vi "Multi-camera acquisition of images.vi"() -> ()   [LabVIEW 2009]
uses:
  D/Program Files (x86)/National Instruments/LabVIEW 2015/user.lib/LabViewDVPCamera/LabViewDVPCamera.lvlib
panel:
  in  "CloseFlg 4":i32
  in  "CameraList 4":u16(ring) caption="CameraList" items=["USB2_1.2M_MONO(31)@UE121000026", "USB3_CMOS_16M(2)@UB16A000000"]
  in  "Set 4":bool
  in  "Open 4":bool
  in  "Close 4":bool
  in  "ScanCamera 4":bool
  out "handle 4":u32
  out "Image 4":T1(plugin-control)
  in  "CloseFlg 3":i32
  in  "CameraList 3":u16(ring) caption="CameraList" items=["USB2_1.2M_MONO(32)@UE121303030", "USB3_CMOS_16M(2)@UB16A000000"]
  in  "Set 3":bool
  in  "Open 3":bool
  in  "Close 3":bool
  in  "ScanCamera 3":bool
  out "handle 3":u32
  out "Image 3":T1(plugin-control)
  in  "CloseFlg 2":i32
  in  "CameraList 2":u16(ring) caption="CameraList" items=["USB2_1.2M_MONO(31)@UE121000026", "USB3_CMOS_16M(2)@UB16A000000"]
  in  "Set 2":bool
  in  "Open 2":bool
  in  "Close 2":bool
  in  "ScanCamera 2":bool
  out "handle 2":u32
  out "Image 2":T1(plugin-control)
  out "Image":T1(plugin-control)
  in  "CloseFlg":i32
  out "handle":u32
  in  "CameraList":u16(ring) items=["USB2_1.2M_MONO(32)@UE121303030", "USB3_CMOS_16M(2)@UB16A000000"]
  in  "Set":bool
  in  "Close":bool
  in  "Open":bool
  in  "ScanCamera":bool
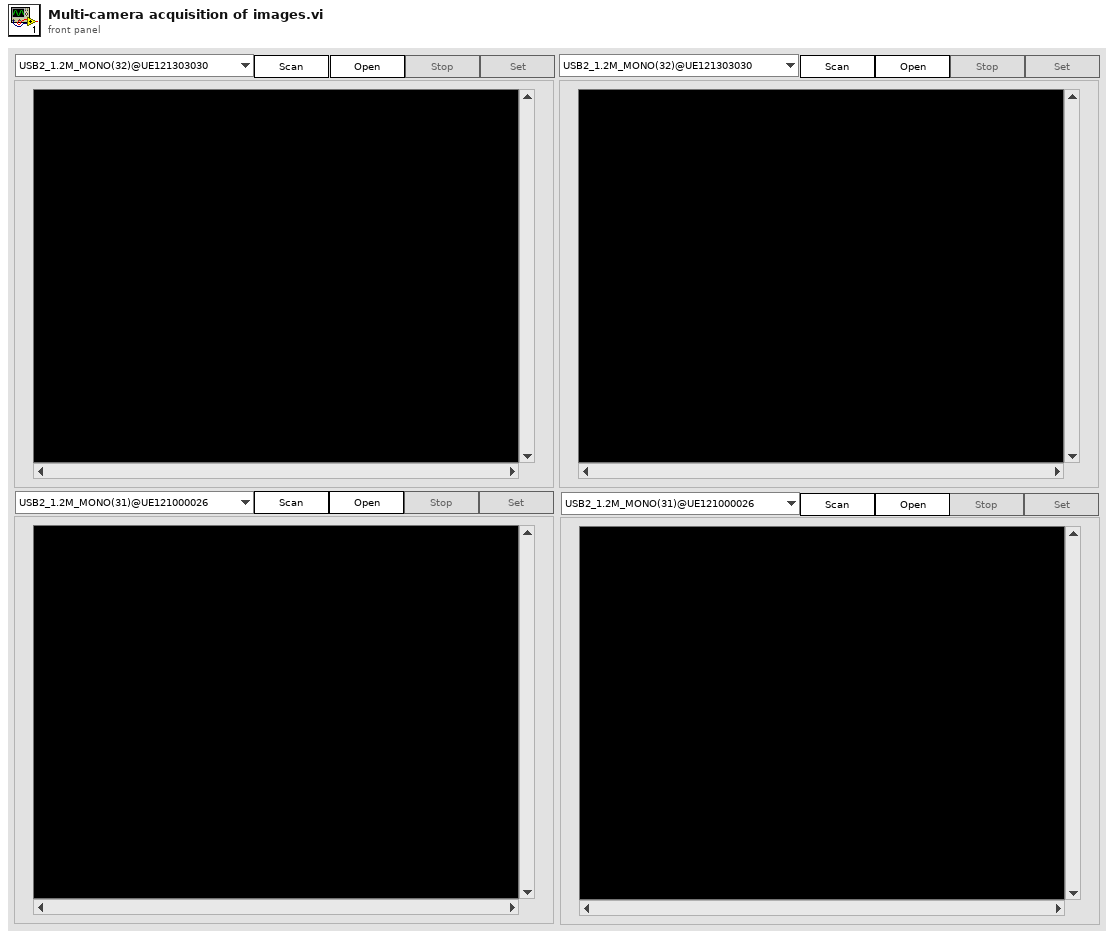
[diagram p1: front panel]
types:
  T1 = typedef "IMAQ Image.ctl" = refnum<image>
  T2 = enum8{"Enabled", "Disabled", "Disabled and Grayed Out"}
  T3 = typedef "LVStringsAndValuesArrayTypeDef_U16.ctl" = cluster{"String":string, "Value":u16}[]
  T4 = typedef "Image Type" = u32
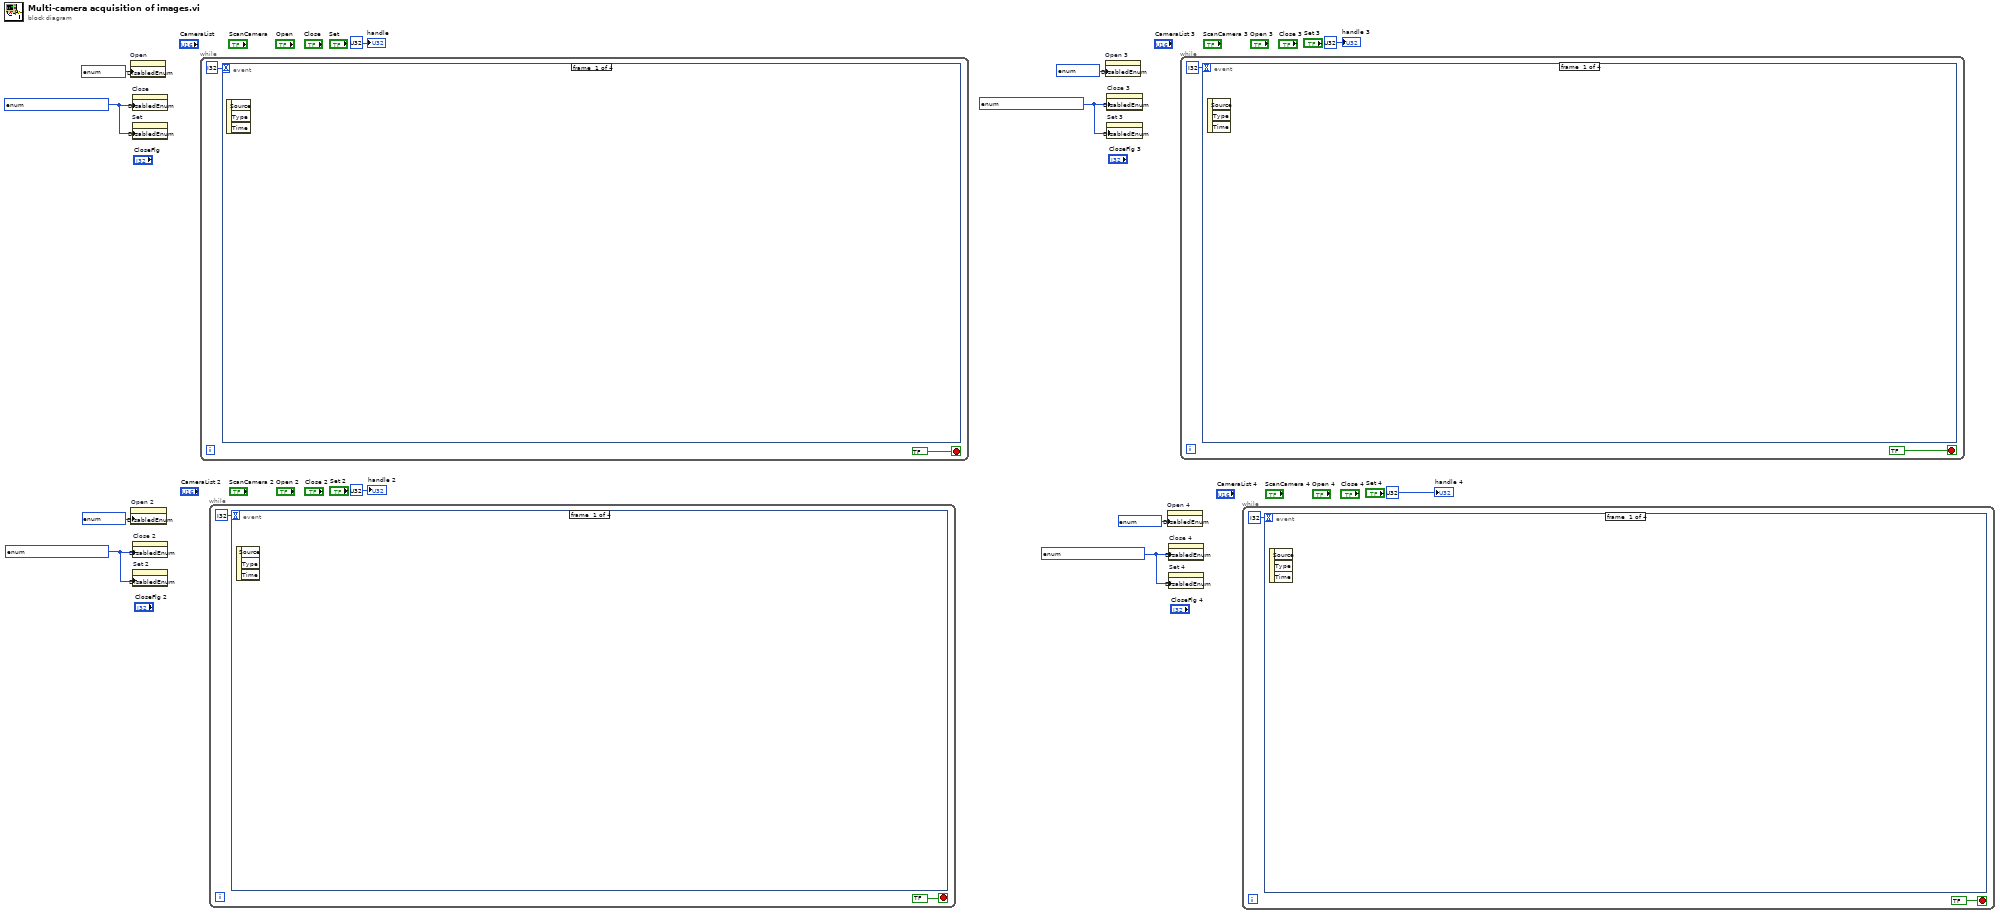
[diagram p0: block diagram]
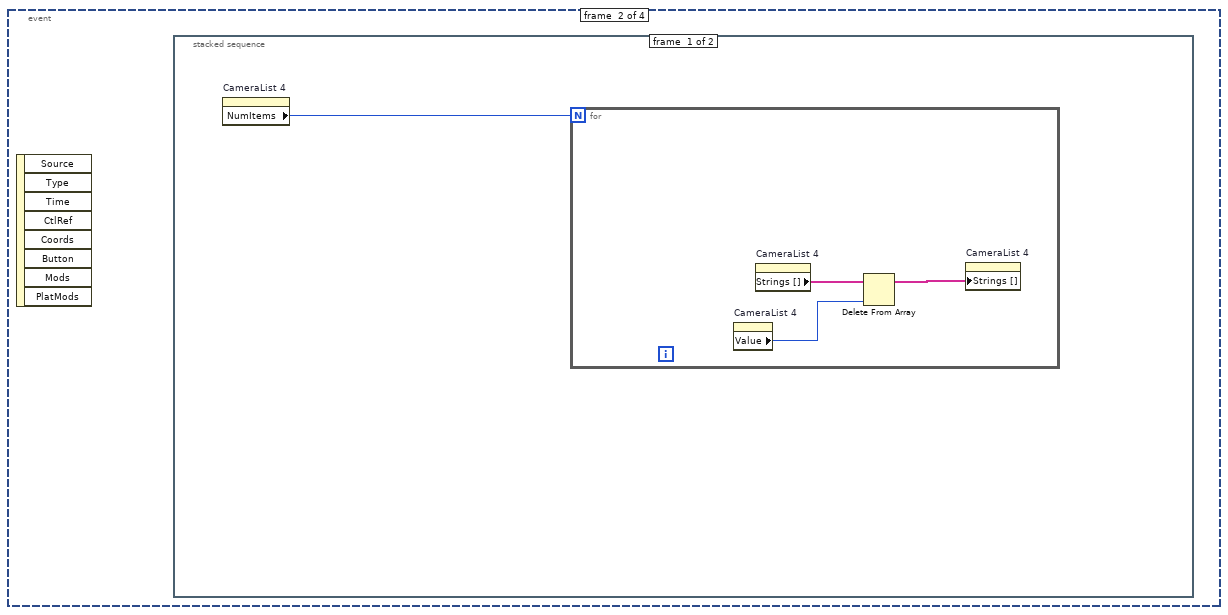
[diagram p2: hidden frame]
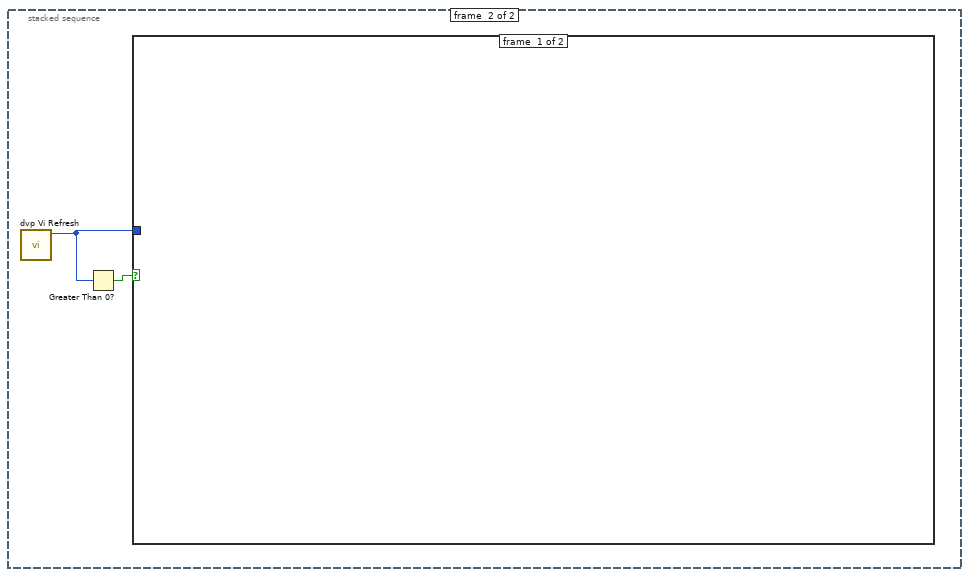
[diagram p3: hidden frame]
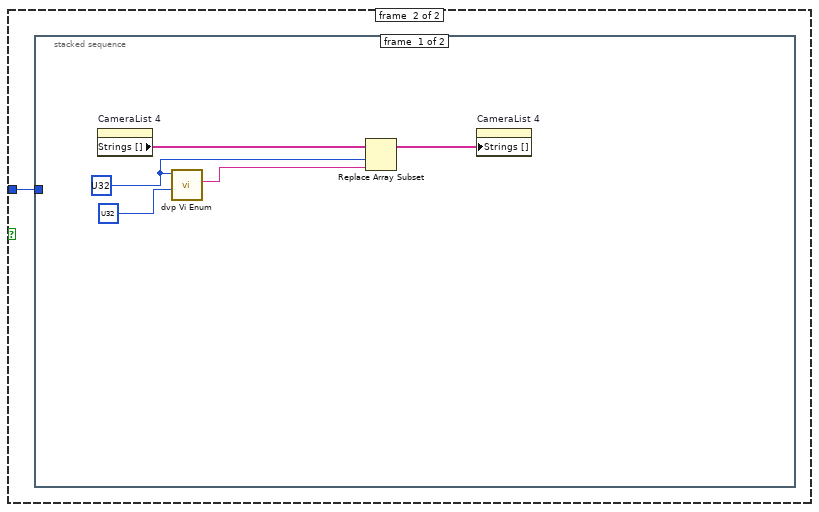
[diagram p4: hidden frame]
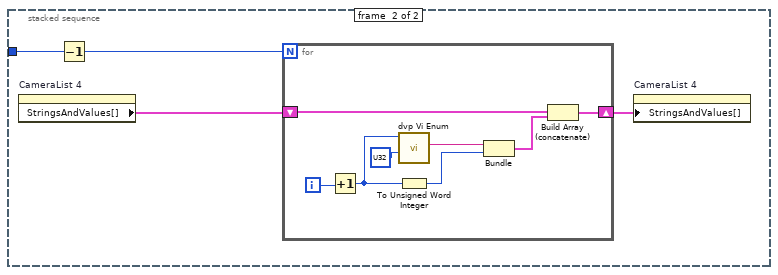
[diagram p5: hidden frame]
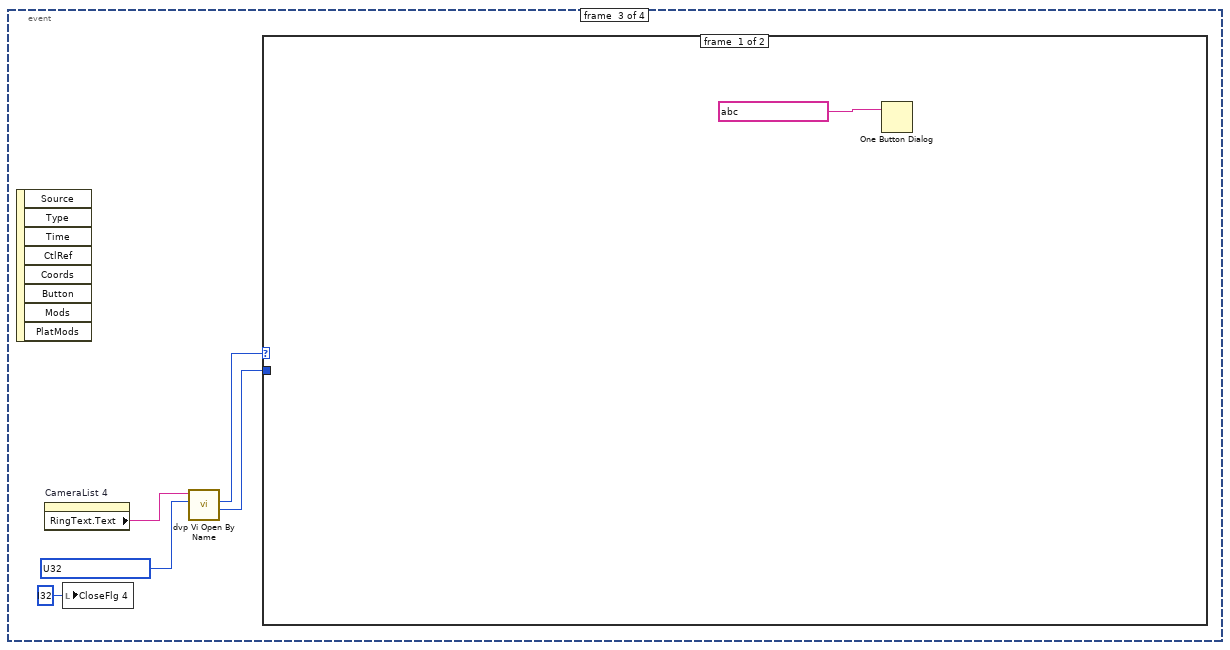
[diagram p6: hidden frame]
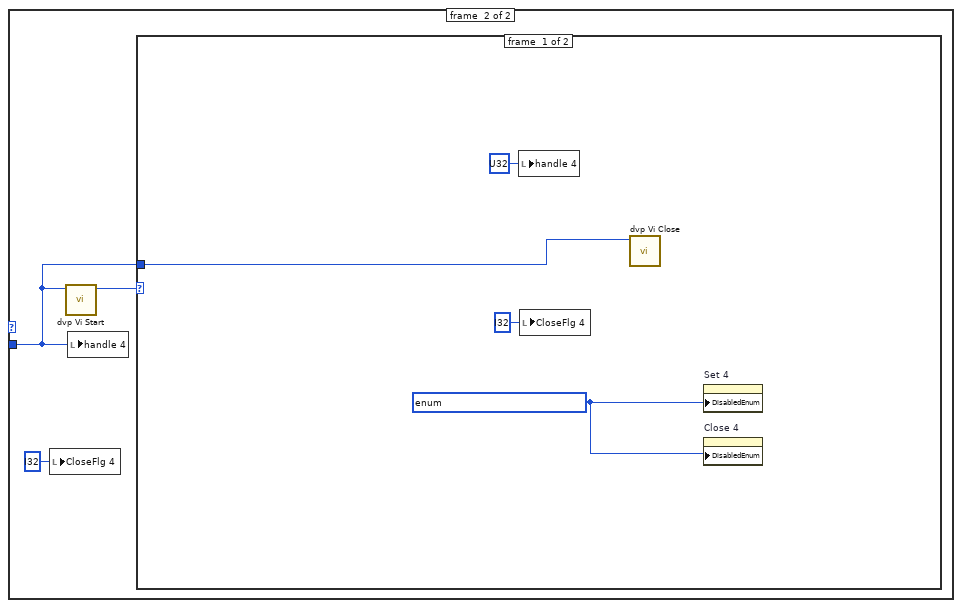
[diagram p7: hidden frame]
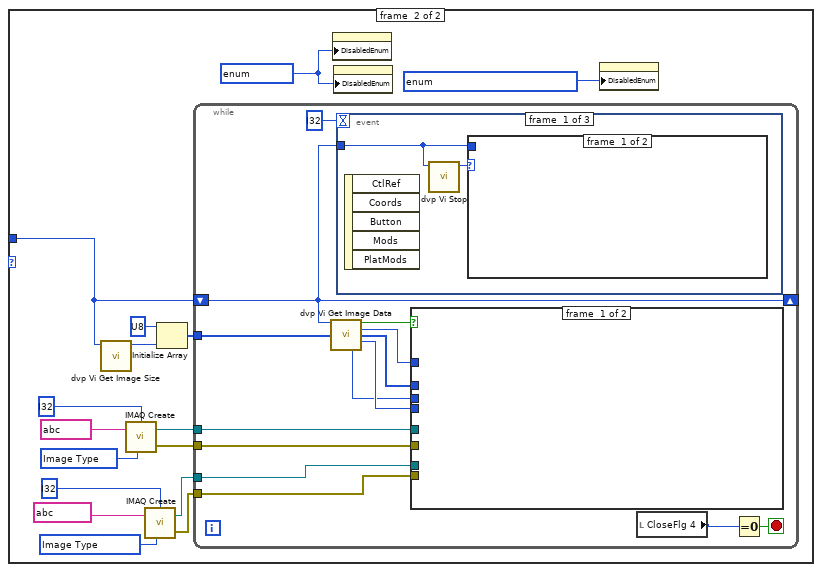
[diagram p8: hidden frame]
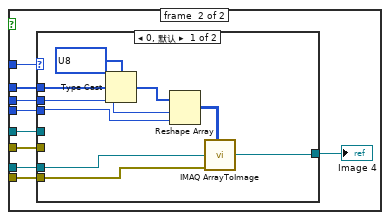
[diagram p9: hidden frame]
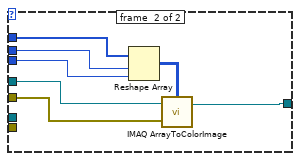
[diagram p10: hidden frame]
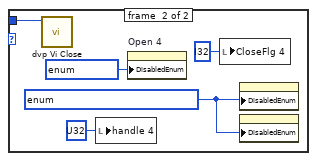
[diagram p11: hidden frame]
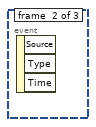
[diagram p12: hidden frame]
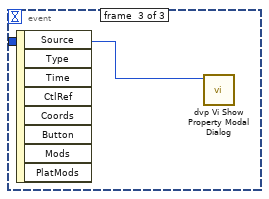
[diagram p13: hidden frame]
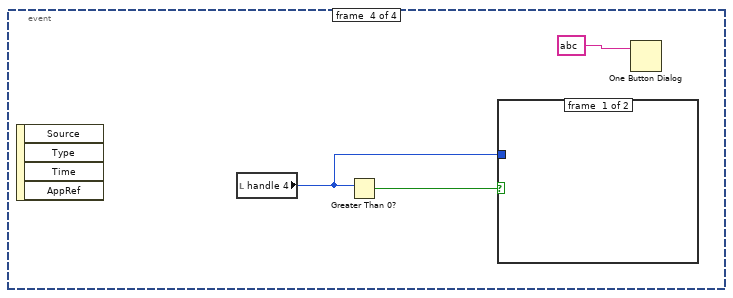
[diagram p14: hidden frame]
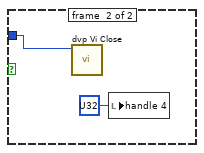
[diagram p15: hidden frame]
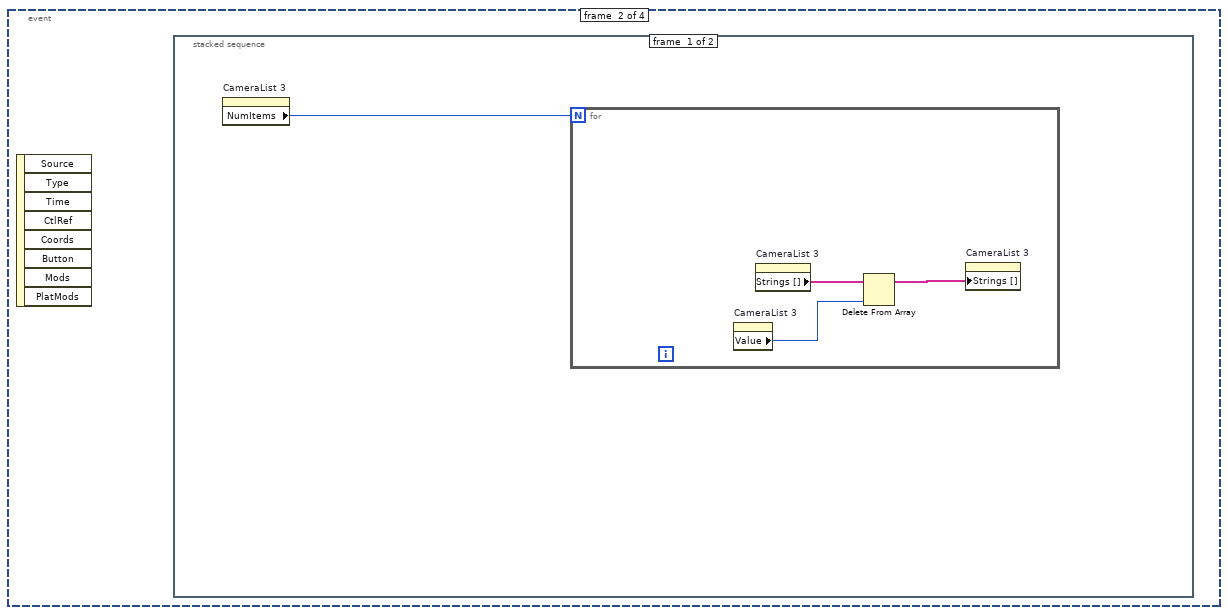
[diagram p16: hidden frame]
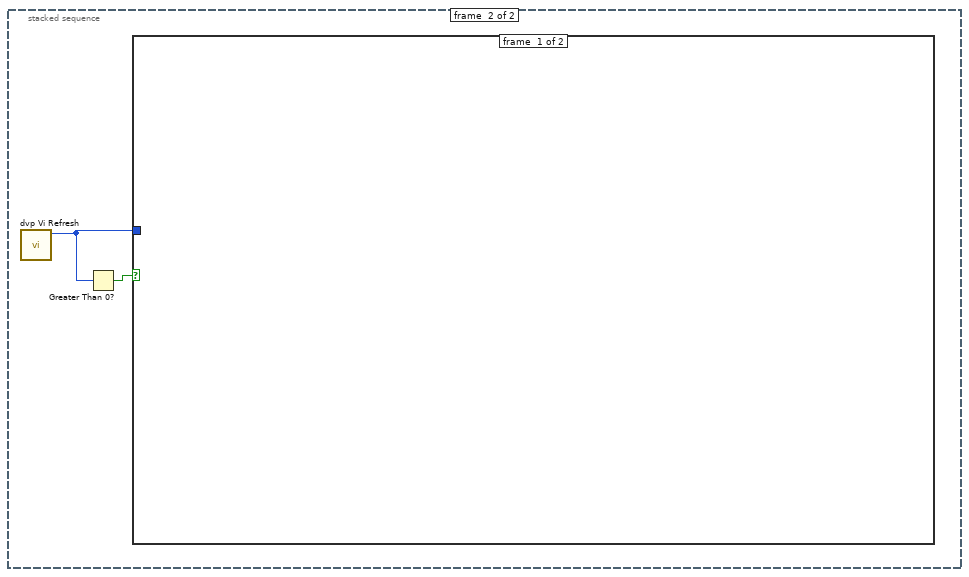
[diagram p17: hidden frame]
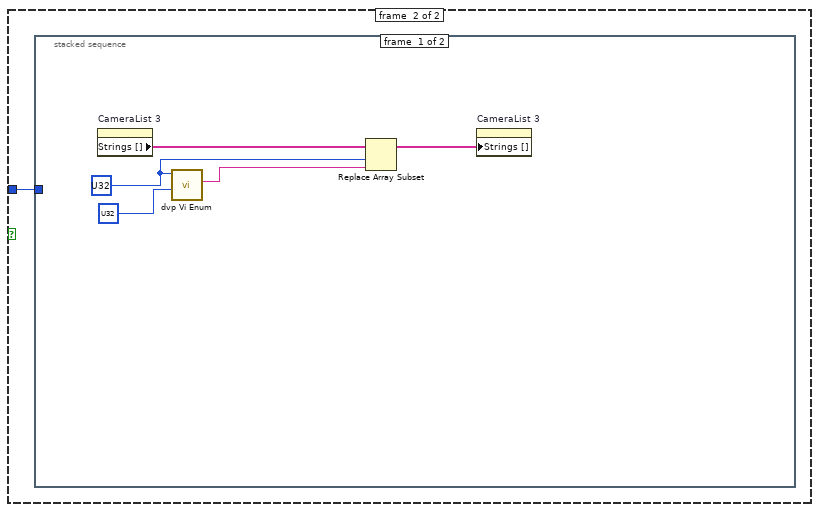
[diagram p18: hidden frame]
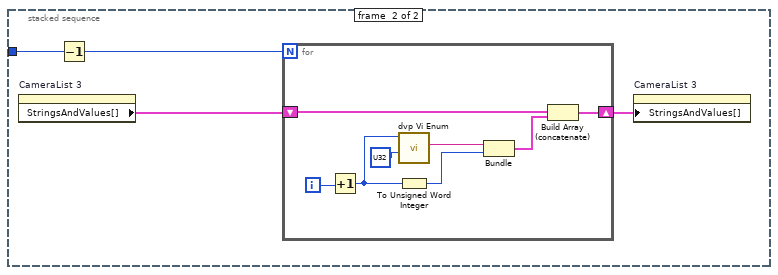
[diagram p19: hidden frame]
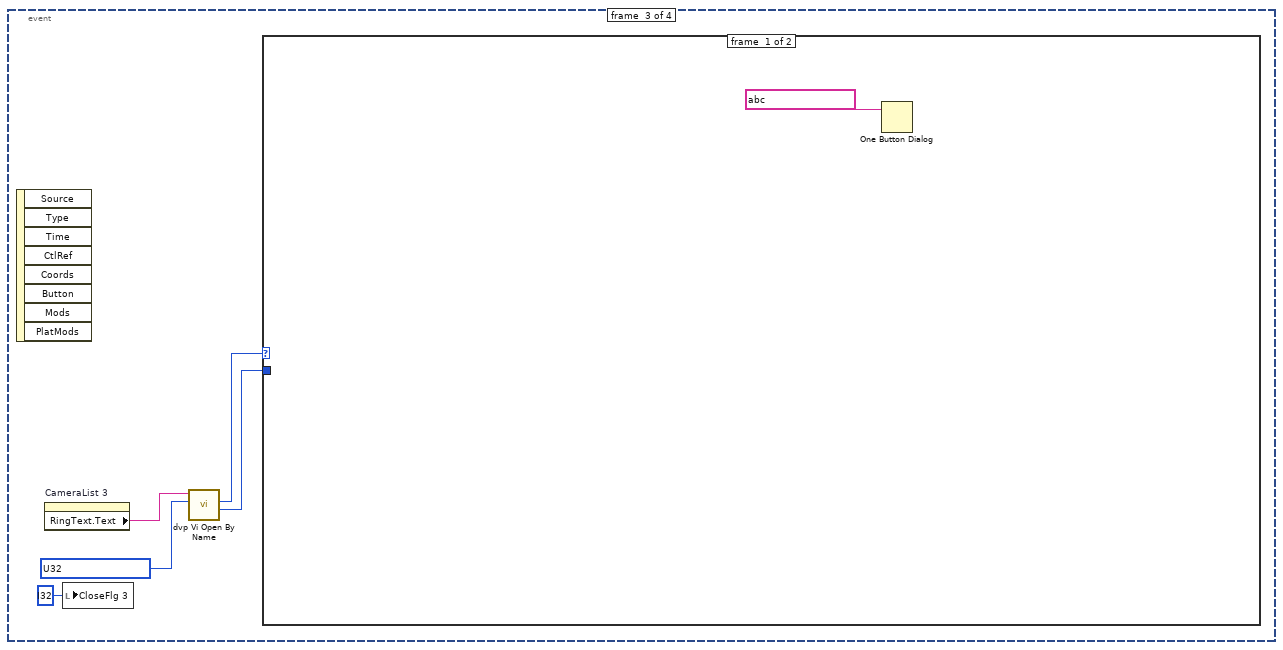
[diagram p20: hidden frame]
diagram:
  w2 = T2 ? ("禁用")
  w5 = T2 ? ("禁用")
  w8 = T2 ? ("禁用")
  w11 = T2 ? ("禁用")
  n1 = property on="Open" class="Bool"("DisabledEnum"=T2 ? ("禁用")) -> ()  [unwired: 2 in, 2 out]
  n2 = property on="Open 2" class="Bool"("DisabledEnum"=T2 ? ("禁用")) -> ()  [unwired: 2 in, 2 out]
  n3 = property on="Close" class="Bool"("DisabledEnum"=w11) -> ()  [unwired: 2 in, 2 out]
  n4 = property on="Set" class="Bool"("DisabledEnum"=w11) -> ()  [unwired: 2 in, 2 out]
  n5 = property on="Close 2" class="Bool"("DisabledEnum"=w8) -> ()  [unwired: 2 in, 2 out]
  n6 = property on="Set 2" class="Bool"("DisabledEnum"=w8) -> ()  [unwired: 2 in, 2 out]
  n7 = while {
    stop <- bool ? stop-if-true
    n8 = event shown="[2] \"Open\": 鼠标按下" {
      selector: _ -> [_ _ _ _]
      dyn-events: _ -> [_ _ _ _]
      timeout: i32 ? -> [_ _ _ _]
      event #0 {
        n9 = event-data() -> ()  [unwired: 1 in, 3 out]
      }
      event #1 {
        n10 = event-data() -> ()  [unwired: 1 in, 8 out]
        n11 = stacked-sequence "清除下拉列表的数据" {
          frame #0 {
            n12 = property on="CameraList" class="Ring (严格)"() -> ("NumItems"=w15:u32)  [unwired: 2 in, 2 out]
            n13 = for {
              N: w15 -> [_]
              n14 = property on="CameraList" class="Ring (严格)"() -> ("Value"=w17:u16)  [unwired: 2 in, 2 out]
              n15 = property on="CameraList" class="Ring (严格)"() -> ("Strings []"=w16:string[])  [unwired: 2 in, 2 out]
              n16 = Delete From Array ("删除数组元素")(array=w16, index=w17) -> (array with subset deleted=w18:string[])  [unwired: 1 in, 1 out]
              n17 = property on="CameraList" class="Ring (严格)"("Strings []"=w18) -> ()  [unwired: 2 in, 2 out]
            }
          }
          frame #1 {
            n18 = call "dvp Vi Refresh.vi"() -> ("pCount out"=w20:u32)  [unwired: 10 in, 1 out]
            n19 = Greater Than 0?(x=w20) -> (x > 0?=w19:bool)
            n20 = case shown="真" w19 {
              tunnel: w20 -> [_ w21]
              frame #0 {
              }
              frame #1 {
                n21 = stacked-sequence {
                  tunnel: w21 -> [_ w28]
                  frame #0 {
                    w22 = u32 ? ("index")
                    n22 = property on="CameraList" class="Ring (严格)"() -> ("Strings []"=w25:string[])  [unwired: 2 in, 2 out]
                    n23 = call "dvp Vi Enum.vi"("unSize"=u32 ?, "index"=w22) -> ("friendlyName out"=w24:string)  [unwired: 8 in, 1 out]
                    n24 = Replace Array Subset ("替换数组子集")(array=w25, new element=w24, index=w22) -> (w26:string[])
                    n25 = property on="CameraList" class="Ring (严格)"("Strings []"=w26) -> ()  [unwired: 2 in, 2 out]
                  }
                  frame #1 {
                    n26 = property on="CameraList" class="Ring (严格)"() -> ("StringsAndValues[]"=w30:T3)  [unwired: 2 in, 2 out]
                    n27 = Decrement(x=w28) -> (x-1=w27:u32)
                    n28 = for {
                      N: w27 -> [_]
                      shift-right: [w37] -> w29
                      shift-left: w30 -> [w35]
                      i -> [w32]
                      n29 = Increment(x=w32) -> (x+1=w31:i32)
                      n30 = call "dvp Vi Enum.vi"("unSize"=u32 ?, "index"=w31) -> ("friendlyName out"=w38:string)  [unwired: 8 in, 1 out]
                      n31 = To Unsigned Word Integer(number=w31) -> (unsigned 16bit integer=w34:u16)
                      n32 = Bundle("friendlyName out"=w38, w34) -> (w36:cluster{"friendlyName out":string, u16})  [unwired: 1 in]
                      n33 = Build Array (concatenate) ("创建数组")(w35, w36) -> (w37:T3)
                    }
                    n34 = property on="CameraList" class="Ring (严格)"("StringsAndValues[]"=w29) -> ()  [unwired: 2 in, 2 out]
                  }
                }
              }
            }
          }
        }
      }
      event #2 {
        w41 = u32 ? items=["OPEN_OFFLINE", "OPEN_NORMAL"] ("type")
        n35 = event-data() -> ()  [unwired: 1 in, 8 out]
        n36 = property on="CameraList" class="Ring (严格)"() -> ("RingText.Text"=w40:string)  [unwired: 2 in, 2 out]
        n37 = local write "CloseFlg"(i32 ? ("CloseFlg")) -> ()
        n38 = call "dvp Vi Open By Name.vi"("type"=w41, "friendlyName"=w40) -> ("pHandle out"=w43:u32, "function return"=w42:u32)  [unwired: 7 in, 1 out]
        n39 = case shown="1" w42 {
          tunnel: w43 -> [_ w47]
          frame #0 {
            n40 = One Button Dialog(message=string ? ("消息")) -> ()  [unwired: 1 in, 1 out]
          }
          frame #1 {
            n41 = call "dvp Vi Start.vi"("handle"=w47) -> ("function return"=w45:u32)  [unwired: 10 in]
            n42 = local write "handle"(w47) -> ()
            n43 = local write "CloseFlg"(i32 ? ("CloseFlg")) -> ()
            n44 = case shown="1" w45 {
              tunnel: w47 -> [w51 w63]
              frame #0 {
                w50 = T2 ? ("禁用")
                n45 = local write "handle"(u32 ? ("handle")) -> ()
                n46 = local write "CloseFlg"(i32 ? ("CloseFlg")) -> ()
                n47 = call "dvp Vi Close.vi"("handle"=w51) -> ()  [unwired: 10 in, 1 out]
                n48 = property on="Set" class="Bool"("DisabledEnum"=w50) -> ()  [unwired: 2 in, 2 out]
                n49 = property on="Close" class="Bool"("DisabledEnum"=w50) -> ()  [unwired: 2 in, 2 out]
              }
              frame #1 {
                w57 = T4 ? items=["Grayscale (U8)", "Grayscale (I16)", "Grayscale (SGL)", "Complex (CSG)", "RGB (U32)", "HSL (U32)", "RGB (U64)", "Grayscale (U16)"] ("Image Type")
                w61 = T4 ? items=["Grayscale (U8)", "Grayscale (I16)", "Grayscale (SGL)", "Complex (CSG)", "RGB (U32)", "HSL (U32)", "RGB (U64)", "Grayscale (U16)"] ("Image Type")
                w67 = T2 ? ("禁用")
                n50 = call "dvp Vi Get Image Size.vi"("handle"=w63) -> ("function return"=w62:u32)  [unwired: 10 in]
                n51 = call "IMAQ Create"("Border Size"=i32 ?, "Image Name"=string ?, "Image Type"=w61) -> ("New Image"=w56:T1, "error out"=w53:errorcluster)  [unwired: 2 in]
                n52 = call "IMAQ Create"("Border Size"=i32 ?, "Image Name"=string ?, "Image Type"=w57) -> ("New Image"=w55:T1, "error out"=w54:errorcluster)  [unwired: 2 in]
                n53 = Initialize Array(u8 ? ("元素"), w62) -> (w64:u8[])
                n54 = while {
                  shift-right: [w78] -> _
                  shift-left: w63 -> [w78]
                  tunnel: w64 -> [w77]
                  tunnel: w56 -> [w71]
                  tunnel: w55 -> [w70]
                  tunnel: w54 -> [w69]
                  tunnel: w53 -> [w68]
                  stop <- w80 stop-if-true
                  n55 = call "dvp Vi Get Image Data.vi"("handle"=w78, "pbuffer"=w77) -> ("piHeight out"=w75:i32, "function return"=w72:bool, "pformat out"=w73:i32, "pbuffer out"=w74:u32[], "piWidth out"=w76:i32)  [unwired: 9 in]
                  n56 = event shown="[0] \"Close\": 鼠标按下" {
                    selector: _ -> [_ _ _]
                    dyn-events: _ -> [_ _ _]
                    timeout: i32 ? -> [_ _ _]
                    tunnel: w78 -> [w107 _ w114]
                    event #0 {
                      n57 = event-data() -> ()  [unwired: 1 in, 5 out]
                      n58 = call "dvp Vi Stop.vi"("handle"=w107) -> ("function return"=w108:u32)  [unwired: 10 in]
                      n59 = case shown="1" w108 {
                        tunnel: w107 -> [_ w111]
                        frame #0 {
                        }
                        frame #1 {
                          w110 = T2 ? ("禁用")
                          n60 = call "dvp Vi Close.vi"("handle"=w111) -> ()  [unwired: 10 in, 1 out]
                          n61 = local write "handle"(u32 ? ("handle")) -> ()
                          n62 = property on="Open" class="Bool"("DisabledEnum"=T2 ? ("禁用")) -> ()  [unwired: 2 in, 2 out]
                          n63 = local write "CloseFlg"(i32 ? ("CloseFlg")) -> ()
                          n64 = property on="Close" class="Bool"("DisabledEnum"=w110) -> ()  [unwired: 2 in, 2 out]
                          n65 = property on="Set" class="Bool"("DisabledEnum"=w110) -> ()  [unwired: 2 in, 2 out]
                        }
                      }
                    }
                    event #1 {
                      n66 = event-data() -> ()  [unwired: 1 in, 3 out]
                    }
                    event #2 {
                      n67 = event-data() -> ()  [unwired: 1 in, 8 out]
                      n68 = call "dvp Vi Show Property Modal Dialog.vi"("handle"=w114) -> ()  [unwired: 10 in, 1 out]
                    }
                  }
                  n69 = case shown="真" w72 {
                    tunnel: w76 -> [_ w90]
                    tunnel: w75 -> [_ w89]
                    tunnel: w74 -> [_ w88]
                    tunnel: w73 -> [_ w87]
                    tunnel: w71 -> [_ w83]
                    tunnel: w70 -> [_ w86]
                    tunnel: w69 -> [_ w85]
                    tunnel: w68 -> [_ w84]
                    frame #0 {
                    }
                    frame #1 {
                      n70 = case shown="1" w87 {
                        tunnel: w89 -> [w99 w105]
                        tunnel: w90 -> [w98 w106]
                        tunnel: [w97 w103] -> w82
                        tunnel: w88 -> [w94 w102]
                        tunnel: w86 -> [w91 _]
                        tunnel: w85 -> [w92 _]
                        tunnel: w84 -> [_ w100]
                        tunnel: w83 -> [_ w101]
                        frame #0 {
                          n71 = Type Cast(type=u8[] ?, x=w94) -> (*(type *) &x=w93:u8[])
                          n72 = Reshape Array ("重排数组维数")(w93, w99, w98) -> (w96:u8[][])
                          n73 = call "IMAQ ArrayToImage"("error in (no error)"=w92, "Image Pixels (U8)"=w96, "Image"=w91) -> ("Image Out"=w97:T1)  [unwired: 7 in, 1 out]
                        }
                        frame #1 {
                          n74 = Reshape Array ("重排数组维数")(w102, w105, w106) -> (w104:u32[][])
                          n75 = call "IMAQ ArrayToColorImage"("Image Pixels (U32)"=w104, "Image"=w101, "error in (no error)"=w100) -> ("Image Out"=w103:T1)  [unwired: 2 in, 1 out]
                        }
                      }
                      "Image" <- w82
                    }
                  }
                  n76 = local read "CloseFlg"() -> (w79:i32)
                  n77 = Equal To 0?(x=w79) -> (x = 0?=w80:bool)
                }
                n78 = property on="Set" class="Bool"("DisabledEnum"=w67) -> ()  [unwired: 2 in, 2 out]
                n79 = property on="Close" class="Bool"("DisabledEnum"=w67) -> ()  [unwired: 2 in, 2 out]
                n80 = property on="Open" class="Bool"("DisabledEnum"=T2 ? ("禁用")) -> ()  [unwired: 2 in, 2 out]
              }
            }
          }
        }
      }
      event #3 {
        n81 = event-data() -> ()  [unwired: 1 in, 4 out]
        n82 = local read "handle"() -> (w115:u32)
        n83 = Greater Than 0?(x=w115) -> (x > 0?=w116:bool)
        n84 = case shown="真" w116 {
          tunnel: w115 -> [_ w119]
          frame #0 {
          }
          frame #1 {
            n85 = call "dvp Vi Close.vi"("handle"=w119) -> ()  [unwired: 10 in, 1 out]
            n86 = local write "handle"(u32 ? ("handle")) -> ()
          }
        }
        n87 = One Button Dialog(message=string ? ("消息")) -> ()  [unwired: 1 in, 1 out]
      }
    }
  }
  n88 = while {
    stop <- bool ? stop-if-true
    n89 = event shown="[2] \"Open 2\": 鼠标按下" {
      selector: _ -> [_ _ _ _]
      dyn-events: _ -> [_ _ _ _]
      timeout: i32 ? -> [_ _ _ _]
      event #0 {
        n90 = event-data() -> ()  [unwired: 1 in, 3 out]
      }
      event #1 {
        n91 = event-data() -> ()  [unwired: 1 in, 8 out]
        n92 = stacked-sequence "清除下拉列表的数据" {
          frame #0 {
            n93 = property on="CameraList 2" class="Ring (严格)"() -> ("NumItems"=w122:u32)  [unwired: 2 in, 2 out]
            n94 = for {
              N: w122 -> [_]
              n95 = property on="CameraList 2" class="Ring (严格)"() -> ("Value"=w124:u16)  [unwired: 2 in, 2 out]
              n96 = property on="CameraList 2" class="Ring (严格)"() -> ("Strings []"=w123:string[])  [unwired: 2 in, 2 out]
              n97 = Delete From Array ("删除数组元素")(array=w123, index=w124) -> (array with subset deleted=w125:string[])  [unwired: 1 in, 1 out]
              n98 = property on="CameraList 2" class="Ring (严格)"("Strings []"=w125) -> ()  [unwired: 2 in, 2 out]
            }
          }
          frame #1 {
            n99 = call "dvp Vi Refresh.vi"() -> ("pCount out"=w127:u32)  [unwired: 10 in, 1 out]
            n100 = Greater Than 0?(x=w127) -> (x > 0?=w126:bool)
            n101 = case shown="真" w126 {
              tunnel: w127 -> [_ w128]
              frame #0 {
              }
              frame #1 {
                n102 = stacked-sequence {
                  tunnel: w128 -> [_ w135]
                  frame #0 {
                    w129 = u32 ? ("index")
                    n103 = property on="CameraList 2" class="Ring (严格)"() -> ("Strings []"=w132:string[])  [unwired: 2 in, 2 out]
                    n104 = call "dvp Vi Enum.vi"("unSize"=u32 ?, "index"=w129) -> ("friendlyName out"=w131:string)  [unwired: 8 in, 1 out]
                    n105 = Replace Array Subset ("替换数组子集")(array=w132, new element=w131, index=w129) -> (w133:string[])
                    n106 = property on="CameraList 2" class="Ring (严格)"("Strings []"=w133) -> ()  [unwired: 2 in, 2 out]
                  }
                  frame #1 {
                    n107 = property on="CameraList 2" class="Ring (严格)"() -> ("StringsAndValues[]"=w137:T3)  [unwired: 2 in, 2 out]
                    n108 = Decrement(x=w135) -> (x-1=w134:u32)
                    n109 = for {
                      N: w134 -> [_]
                      shift-right: [w144] -> w136
                      shift-left: w137 -> [w142]
                      i -> [w139]
                      n110 = Increment(x=w139) -> (x+1=w138:i32)
                      n111 = call "dvp Vi Enum.vi"("unSize"=u32 ?, "index"=w138) -> ("friendlyName out"=w145:string)  [unwired: 8 in, 1 out]
                      n112 = To Unsigned Word Integer(number=w138) -> (unsigned 16bit integer=w141:u16)
                      n113 = Bundle("friendlyName out"=w145, w141) -> (w143:cluster{"friendlyName out":string, u16})  [unwired: 1 in]
                      n114 = Build Array (concatenate) ("创建数组")(w142, w143) -> (w144:T3)
                    }
                    n115 = property on="CameraList 2" class="Ring (严格)"("StringsAndValues[]"=w136) -> ()  [unwired: 2 in, 2 out]
                  }
                }
              }
            }
          }
        }
      }
      event #2 {
        w148 = u32 ? items=["OPEN_OFFLINE", "OPEN_NORMAL"] ("type")
        n116 = event-data() -> ()  [unwired: 1 in, 8 out]
        n117 = property on="CameraList 2" class="Ring (严格)"() -> ("RingText.Text"=w147:string)  [unwired: 2 in, 2 out]
        n118 = local write "CloseFlg 2"(i32 ? ("CloseFlg")) -> ()
        n119 = call "dvp Vi Open By Name.vi"("type"=w148, "friendlyName"=w147) -> ("pHandle out"=w150:u32, "function return"=w149:u32)  [unwired: 7 in, 1 out]
        n120 = case shown="1" w149 {
          tunnel: w150 -> [_ w154]
          frame #0 {
            n121 = One Button Dialog(message=string ? ("消息")) -> ()  [unwired: 1 in, 1 out]
          }
          frame #1 {
            n122 = local write "CloseFlg 2"(i32 ? ("CloseFlg")) -> ()
            n123 = call "dvp Vi Start.vi"("handle"=w154) -> ("function return"=w152:u32)  [unwired: 10 in]
            n124 = local write "handle 2"(w154) -> ()
            n125 = case shown="1" w152 {
              tunnel: w154 -> [w158 w170]
              frame #0 {
                w157 = T2 ? ("禁用")
                n126 = local write "handle 2"(u32 ? ("handle")) -> ()
                n127 = local write "CloseFlg 2"(i32 ? ("CloseFlg")) -> ()
                n128 = call "dvp Vi Close.vi"("handle"=w158) -> ()  [unwired: 10 in, 1 out]
                n129 = property on="Set 2" class="Bool"("DisabledEnum"=w157) -> ()  [unwired: 2 in, 2 out]
                n130 = property on="Close 2" class="Bool"("DisabledEnum"=w157) -> ()  [unwired: 2 in, 2 out]
              }
              frame #1 {
                w165 = T4 ? items=["Grayscale (U8)", "Grayscale (I16)", "Grayscale (SGL)", "Complex (CSG)", "RGB (U32)", "HSL (U32)", "RGB (U64)", "Grayscale (U16)"] ("Image Type")
                w168 = T4 ? items=["Grayscale (U8)", "Grayscale (I16)", "Grayscale (SGL)", "Complex (CSG)", "RGB (U32)", "HSL (U32)", "RGB (U64)", "Grayscale (U16)"] ("Image Type")
                w174 = T2 ? ("禁用")
                n131 = call "dvp Vi Get Image Size.vi"("handle"=w170) -> ("function return"=w169:u32)  [unwired: 10 in]
                n132 = call "IMAQ Create"("Border Size"=i32 ?, "Image Name"=string ?, "Image Type"=w165) -> ("New Image"=w162:T1, "error out"=w161:errorcluster)  [unwired: 2 in]
                n133 = call "IMAQ Create"("Border Size"=i32 ?, "Image Name"=string ?, "Image Type"=w168) -> ("New Image"=w160:T1, "error out"=w159:errorcluster)  [unwired: 2 in]
                n134 = Initialize Array(u8 ? ("元素"), w169) -> (w171:u8[])
                n135 = while {
                  shift-right: [w185] -> _
                  shift-left: w170 -> [w185]
                  tunnel: w171 -> [w184]
                  tunnel: w162 -> [w178]
                  tunnel: w161 -> [w177]
                  tunnel: w160 -> [w176]
                  tunnel: w159 -> [w175]
                  stop <- w187 stop-if-true
                  n136 = call "dvp Vi Get Image Data.vi"("handle"=w185, "pbuffer"=w184) -> ("piHeight out"=w182:i32, "function return"=w179:bool, "pformat out"=w180:i32, "pbuffer out"=w181:u32[], "piWidth out"=w183:i32)  [unwired: 9 in]
                  n137 = event shown="[2] \"Set 2\": 鼠标按下" {
                    selector: _ -> [_ _ _]
                    dyn-events: _ -> [_ _ _]
                    timeout: i32 ? -> [_ _ _]
                    tunnel: w185 -> [w214 _ w221]
                    event #0 {
                      n138 = event-data() -> ()  [unwired: 1 in, 5 out]
                      n139 = call "dvp Vi Stop.vi"("handle"=w214) -> ("function return"=w215:u32)  [unwired: 10 in]
                      n140 = case shown="1" w215 {
                        tunnel: w214 -> [_ w218]
                        frame #0 {
                        }
                        frame #1 {
                          w217 = T2 ? ("禁用")
                          n141 = call "dvp Vi Close.vi"("handle"=w218) -> ()  [unwired: 10 in, 1 out]
                          n142 = local write "handle 2"(u32 ? ("handle")) -> ()
                          n143 = property on="Open 2" class="Bool"("DisabledEnum"=T2 ? ("禁用")) -> ()  [unwired: 2 in, 2 out]
                          n144 = local write "CloseFlg 2"(i32 ? ("CloseFlg")) -> ()
                          n145 = property on="Close 2" class="Bool"("DisabledEnum"=w217) -> ()  [unwired: 2 in, 2 out]
                          n146 = property on="Set 2" class="Bool"("DisabledEnum"=w217) -> ()  [unwired: 2 in, 2 out]
                        }
                      }
                    }
                    event #1 {
                      n147 = event-data() -> ()  [unwired: 1 in, 3 out]
                    }
                    event #2 {
                      n148 = event-data() -> ()  [unwired: 1 in, 8 out]
                      n149 = call "dvp Vi Show Property Modal Dialog.vi"("handle"=w221) -> ()  [unwired: 10 in, 1 out]
                    }
                  }
                  n150 = case shown="真" w179 {
                    tunnel: w183 -> [_ w197]
                    tunnel: w182 -> [_ w196]
                    tunnel: w181 -> [_ w194]
                    tunnel: w180 -> [_ w193]
                    tunnel: w178 -> [_ w192]
                    tunnel: w177 -> [_ w191]
                    tunnel: w176 -> [_ w190]
                    tunnel: w175 -> [_ w189]
                    frame #0 {
                    }
                    frame #1 {
                      n151 = case shown="0, 默认" w193 {
                        tunnel: w196 -> [w206 w212]
                        tunnel: w197 -> [w205 w213]
                        tunnel: [w204 w210] -> w195
                        tunnel: w194 -> [w201 w209]
                        tunnel: w192 -> [_ w208]
                        tunnel: w191 -> [_ w207]
                        tunnel: w190 -> [w198 _]
                        tunnel: w189 -> [w199 _]
                        frame #0 {
                          n152 = Type Cast(type=u8[] ?, x=w201) -> (*(type *) &x=w200:u8[])
                          n153 = Reshape Array ("重排数组维数")(w200, w206, w205) -> (w203:u8[][])
                          n154 = call "IMAQ ArrayToImage"("error in (no error)"=w199, "Image Pixels (U8)"=w203, "Image"=w198) -> ("Image Out"=w204:T1)  [unwired: 7 in, 1 out]
                        }
                        frame #1 {
                          n155 = Reshape Array ("重排数组维数")(w209, w212, w213) -> (w211:u32[][])
                          n156 = call "IMAQ ArrayToColorImage"("Image Pixels (U32)"=w211, "Image"=w208, "error in (no error)"=w207) -> ("Image Out"=w210:T1)  [unwired: 2 in, 1 out]
                        }
                      }
                      "Image 2" <- w195
                    }
                  }
                  n157 = local read "CloseFlg 2"() -> (w186:i32)
                  n158 = Equal To 0?(x=w186) -> (x = 0?=w187:bool)
                }
                n159 = property on="Set 2" class="Bool"("DisabledEnum"=w174) -> ()  [unwired: 2 in, 2 out]
                n160 = property on="Close 2" class="Bool"("DisabledEnum"=w174) -> ()  [unwired: 2 in, 2 out]
                n161 = property on="Open 2" class="Bool"("DisabledEnum"=T2 ? ("禁用")) -> ()  [unwired: 2 in, 2 out]
              }
            }
          }
        }
      }
      event #3 {
        n162 = event-data() -> ()  [unwired: 1 in, 4 out]
        n163 = local read "handle 2"() -> (w222:u32)
        n164 = Greater Than 0?(x=w222) -> (x > 0?=w223:bool)
        n165 = case shown="真" w223 {
          tunnel: w222 -> [_ w226]
          frame #0 {
          }
          frame #1 {
            n166 = call "dvp Vi Close.vi"("handle"=w226) -> ()  [unwired: 10 in, 1 out]
            n167 = local write "handle 2"(u32 ? ("handle")) -> ()
          }
        }
        n168 = One Button Dialog(message=string ? ("消息")) -> ()  [unwired: 1 in, 1 out]
      }
    }
  }
  n169 = property on="Open 3" class="Bool"("DisabledEnum"=T2 ? ("禁用")) -> ()  [unwired: 2 in, 2 out]
  n170 = property on="Close 3" class="Bool"("DisabledEnum"=w5) -> ()  [unwired: 2 in, 2 out]
  n171 = property on="Set 3" class="Bool"("DisabledEnum"=w5) -> ()  [unwired: 2 in, 2 out]
  n172 = property on="Open 4" class="Bool"("DisabledEnum"=T2 ? ("禁用")) -> ()  [unwired: 2 in, 2 out]
  n173 = property on="Close 4" class="Bool"("DisabledEnum"=w2) -> ()  [unwired: 2 in, 2 out]
  n174 = property on="Set 4" class="Bool"("DisabledEnum"=w2) -> ()  [unwired: 2 in, 2 out]
  n175 = while {
    stop <- bool ? stop-if-true
    n176 = event shown="[1] \"ScanCamera 3\": 鼠标按下" {
      selector: _ -> [_ _ _ _]
      dyn-events: _ -> [_ _ _ _]
      timeout: i32 ? -> [_ _ _ _]
      event #0 {
        n177 = event-data() -> ()  [unwired: 1 in, 3 out]
      }
      event #1 {
        n178 = event-data() -> ()  [unwired: 1 in, 8 out]
        n179 = stacked-sequence "清除下拉列表的数据" {
          frame #0 {
            n180 = property on="CameraList 3" class="Ring (严格)"() -> ("NumItems"=w229:u32)  [unwired: 2 in, 2 out]
            n181 = for {
              N: w229 -> [_]
              n182 = property on="CameraList 3" class="Ring (严格)"() -> ("Value"=w231:u16)  [unwired: 2 in, 2 out]
              n183 = property on="CameraList 3" class="Ring (严格)"() -> ("Strings []"=w230:string[])  [unwired: 2 in, 2 out]
              n184 = Delete From Array ("删除数组元素")(array=w230, index=w231) -> (array with subset deleted=w232:string[])  [unwired: 1 in, 1 out]
              n185 = property on="CameraList 3" class="Ring (严格)"("Strings []"=w232) -> ()  [unwired: 2 in, 2 out]
            }
          }
          frame #1 {
            n186 = call "dvp Vi Refresh.vi"() -> ("pCount out"=w234:u32)  [unwired: 10 in, 1 out]
            n187 = Greater Than 0?(x=w234) -> (x > 0?=w233:bool)
            n188 = case shown="真" w233 {
              tunnel: w234 -> [_ w235]
              frame #0 {
              }
              frame #1 {
                n189 = stacked-sequence {
                  tunnel: w235 -> [_ w242]
                  frame #0 {
                    w236 = u32 ? ("index")
                    n190 = property on="CameraList 3" class="Ring (严格)"() -> ("Strings []"=w239:string[])  [unwired: 2 in, 2 out]
                    n191 = call "dvp Vi Enum.vi"("unSize"=u32 ?, "index"=w236) -> ("friendlyName out"=w238:string)  [unwired: 8 in, 1 out]
                    n192 = Replace Array Subset ("替换数组子集")(array=w239, new element=w238, index=w236) -> (w240:string[])
                    n193 = property on="CameraList 3" class="Ring (严格)"("Strings []"=w240) -> ()  [unwired: 2 in, 2 out]
                  }
                  frame #1 {
                    n194 = property on="CameraList 3" class="Ring (严格)"() -> ("StringsAndValues[]"=w244:T3)  [unwired: 2 in, 2 out]
                    n195 = Decrement(x=w242) -> (x-1=w241:u32)
                    n196 = for {
                      N: w241 -> [_]
                      shift-right: [w251] -> w243
                      shift-left: w244 -> [w249]
                      i -> [w246]
                      n197 = Increment(x=w246) -> (x+1=w245:i32)
                      n198 = call "dvp Vi Enum.vi"("unSize"=u32 ?, "index"=w245) -> ("friendlyName out"=w252:string)  [unwired: 8 in, 1 out]
                      n199 = To Unsigned Word Integer(number=w245) -> (unsigned 16bit integer=w248:u16)
                      n200 = Bundle("friendlyName out"=w252, w248) -> (w250:cluster{"friendlyName out":string, u16})  [unwired: 1 in]
                      n201 = Build Array (concatenate) ("创建数组")(w249, w250) -> (w251:T3)
                    }
                    n202 = property on="CameraList 3" class="Ring (严格)"("StringsAndValues[]"=w243) -> ()  [unwired: 2 in, 2 out]
                  }
                }
              }
            }
          }
        }
      }
      event #2 {
        w255 = u32 ? items=["OPEN_OFFLINE", "OPEN_NORMAL"] ("type")
        n203 = event-data() -> ()  [unwired: 1 in, 8 out]
        n204 = property on="CameraList 3" class="Ring (严格)"() -> ("RingText.Text"=w254:string)  [unwired: 2 in, 2 out]
        n205 = local write "CloseFlg 3"(i32 ? ("CloseFlg")) -> ()
        n206 = call "dvp Vi Open By Name.vi"("type"=w255, "friendlyName"=w254) -> ("pHandle out"=w257:u32, "function return"=w256:u32)  [unwired: 7 in, 1 out]
        n207 = case shown="1" w256 {
          tunnel: w257 -> [_ w261]
          frame #0 {
            n208 = One Button Dialog(message=string ? ("消息")) -> ()  [unwired: 1 in, 1 out]
          }
          frame #1 {
            n209 = local write "CloseFlg 3"(i32 ? ("CloseFlg")) -> ()
            n210 = call "dvp Vi Start.vi"("handle"=w261) -> ("function return"=w259:u32)  [unwired: 10 in]
            n211 = local write "handle 3"(w261) -> ()
            n212 = case shown="1" w259 {
              tunnel: w261 -> [w265 w277]
              frame #0 {
                w264 = T2 ? ("禁用")
                n213 = local write "handle 3"(u32 ? ("handle")) -> ()
                n214 = local write "CloseFlg 3"(i32 ? ("CloseFlg")) -> ()
                n215 = call "dvp Vi Close.vi"("handle"=w265) -> ()  [unwired: 10 in, 1 out]
                n216 = property on="Set 3" class="Bool"("DisabledEnum"=w264) -> ()  [unwired: 2 in, 2 out]
                n217 = property on="Close 3" class="Bool"("DisabledEnum"=w264) -> ()  [unwired: 2 in, 2 out]
              }
              frame #1 {
                w273 = T4 ? items=["Grayscale (U8)", "Grayscale (I16)", "Grayscale (SGL)", "Complex (CSG)", "RGB (U32)", "HSL (U32)", "RGB (U64)", "Grayscale (U16)"] ("Image Type")
                w275 = T4 ? items=["Grayscale (U8)", "Grayscale (I16)", "Grayscale (SGL)", "Complex (CSG)", "RGB (U32)", "HSL (U32)", "RGB (U64)", "Grayscale (U16)"] ("Image Type")
                w281 = T2 ? ("禁用")
                n218 = call "dvp Vi Get Image Size.vi"("handle"=w277) -> ("function return"=w276:u32)  [unwired: 10 in]
                n219 = call "IMAQ Create"("Border Size"=i32 ?, "Image Name"=string ?, "Image Type"=w275) -> ("New Image"=w267:T1, "error out"=w266:errorcluster)  [unwired: 2 in]
                n220 = call "IMAQ Create"("Border Size"=i32 ?, "Image Name"=string ?, "Image Type"=w273) -> ("New Image"=w269:T1, "error out"=w268:errorcluster)  [unwired: 2 in]
                n221 = Initialize Array(u8 ? ("元素"), w276) -> (w278:u8[])
                n222 = while {
                  shift-right: [w292] -> _
                  shift-left: w277 -> [w292]
                  tunnel: w278 -> [w291]
                  tunnel: w269 -> [w285]
                  tunnel: w268 -> [w284]
                  tunnel: w267 -> [w283]
                  tunnel: w266 -> [w282]
                  stop <- w294 stop-if-true
                  n223 = call "dvp Vi Get Image Data.vi"("handle"=w292, "pbuffer"=w291) -> ("piHeight out"=w289:i32, "function return"=w286:bool, "pformat out"=w287:i32, "pbuffer out"=w288:u32[], "piWidth out"=w290:i32)  [unwired: 9 in]
                  n224 = event shown="[2] \"Set 3\": 鼠标按下" {
                    selector: _ -> [_ _ _]
                    dyn-events: _ -> [_ _ _]
                    timeout: i32 ? -> [_ _ _]
                    tunnel: w292 -> [w321 _ w328]
                    event #0 {
                      n225 = event-data() -> ()  [unwired: 1 in, 5 out]
                      n226 = call "dvp Vi Stop.vi"("handle"=w321) -> ("function return"=w322:u32)  [unwired: 10 in]
                      n227 = case shown="1" w322 {
                        tunnel: w321 -> [_ w325]
                        frame #0 {
                        }
                        frame #1 {
                          w324 = T2 ? ("禁用")
                          n228 = call "dvp Vi Close.vi"("handle"=w325) -> ()  [unwired: 10 in, 1 out]
                          n229 = local write "handle 3"(u32 ? ("handle")) -> ()
                          n230 = property on="Open 3" class="Bool"("DisabledEnum"=T2 ? ("禁用")) -> ()  [unwired: 2 in, 2 out]
                          n231 = local write "CloseFlg 3"(i32 ? ("CloseFlg")) -> ()
                          n232 = property on="Close 3" class="Bool"("DisabledEnum"=w324) -> ()  [unwired: 2 in, 2 out]
                          n233 = property on="Set 3" class="Bool"("DisabledEnum"=w324) -> ()  [unwired: 2 in, 2 out]
                        }
                      }
                    }
                    event #1 {
                      n234 = event-data() -> ()  [unwired: 1 in, 3 out]
                    }
                    event #2 {
                      n235 = event-data() -> ()  [unwired: 1 in, 8 out]
                      n236 = call "dvp Vi Show Property Modal Dialog.vi"("handle"=w328) -> ()  [unwired: 10 in, 1 out]
                    }
                  }
                  n237 = case shown="真" w286 {
                    tunnel: w290 -> [_ w304]
                    tunnel: w289 -> [_ w303]
                    tunnel: w288 -> [_ w302]
                    tunnel: w287 -> [_ w301]
                    tunnel: w285 -> [_ w300]
                    tunnel: w284 -> [_ w299]
                    tunnel: w283 -> [_ w298]
                    tunnel: w282 -> [_ w297]
                    frame #0 {
                    }
                    frame #1 {
                      n238 = case shown="1" w301 {
                        tunnel: w303 -> [w313 w319]
                        tunnel: w304 -> [w312 w320]
                        tunnel: [w311 w317] -> w296
                        tunnel: w302 -> [w308 w316]
                        tunnel: w300 -> [w306 _]
                        tunnel: w299 -> [w305 _]
                        tunnel: w298 -> [_ w315]
                        tunnel: w297 -> [_ w314]
                        frame #0 {
                          n239 = Type Cast(type=u8[] ?, x=w308) -> (*(type *) &x=w307:u8[])
                          n240 = Reshape Array ("重排数组维数")(w307, w313, w312) -> (w310:u8[][])
                          n241 = call "IMAQ ArrayToImage"("error in (no error)"=w305, "Image Pixels (U8)"=w310, "Image"=w306) -> ("Image Out"=w311:T1)  [unwired: 7 in, 1 out]
                        }
                        frame #1 {
                          n242 = Reshape Array ("重排数组维数")(w316, w319, w320) -> (w318:u32[][])
                          n243 = call "IMAQ ArrayToColorImage"("Image Pixels (U32)"=w318, "Image"=w315, "error in (no error)"=w314) -> ("Image Out"=w317:T1)  [unwired: 2 in, 1 out]
                        }
                      }
                      "Image 3" <- w296
                    }
                  }
                  n244 = local read "CloseFlg 3"() -> (w293:i32)
                  n245 = Equal To 0?(x=w293) -> (x = 0?=w294:bool)
                }
                n246 = property on="Set 3" class="Bool"("DisabledEnum"=w281) -> ()  [unwired: 2 in, 2 out]
                n247 = property on="Close 3" class="Bool"("DisabledEnum"=w281) -> ()  [unwired: 2 in, 2 out]
                n248 = property on="Open 3" class="Bool"("DisabledEnum"=T2 ? ("禁用")) -> ()  [unwired: 2 in, 2 out]
              }
            }
          }
        }
      }
      event #3 {
        n249 = event-data() -> ()  [unwired: 1 in, 4 out]
        n250 = local read "handle 3"() -> (w329:u32)
        n251 = Greater Than 0?(x=w329) -> (x > 0?=w330:bool)
        n252 = case shown="真" w330 {
          tunnel: w329 -> [_ w333]
          frame #0 {
          }
          frame #1 {
            n253 = call "dvp Vi Close.vi"("handle"=w333) -> ()  [unwired: 10 in, 1 out]
            n254 = local write "handle 3"(u32 ? ("handle")) -> ()
          }
        }
        n255 = One Button Dialog(message=string ? ("消息")) -> ()  [unwired: 1 in, 1 out]
      }
    }
  }
  n256 = while {
    stop <- bool ? stop-if-true
    n257 = event shown="[2] \"Open 4\": 鼠标按下" {
      selector: _ -> [_ _ _ _]
      dyn-events: _ -> [_ _ _ _]
      timeout: i32 ? -> [_ _ _ _]
      event #0 {
        n258 = event-data() -> ()  [unwired: 1 in, 3 out]
      }
      event #1 {
        n259 = event-data() -> ()  [unwired: 1 in, 8 out]
        n260 = stacked-sequence "清除下拉列表的数据" {
          frame #0 {
            n261 = property on="CameraList 4" class="Ring (严格)"() -> ("NumItems"=w336:u32)  [unwired: 2 in, 2 out]
            n262 = for {
              N: w336 -> [_]
              n263 = property on="CameraList 4" class="Ring (严格)"() -> ("Value"=w338:u16)  [unwired: 2 in, 2 out]
              n264 = property on="CameraList 4" class="Ring (严格)"() -> ("Strings []"=w337:string[])  [unwired: 2 in, 2 out]
              n265 = Delete From Array ("删除数组元素")(array=w337, index=w338) -> (array with subset deleted=w339:string[])  [unwired: 1 in, 1 out]
              n266 = property on="CameraList 4" class="Ring (严格)"("Strings []"=w339) -> ()  [unwired: 2 in, 2 out]
            }
          }
          frame #1 {
            n267 = call "dvp Vi Refresh.vi"() -> ("pCount out"=w341:u32)  [unwired: 10 in, 1 out]
            n268 = Greater Than 0?(x=w341) -> (x > 0?=w340:bool)
            n269 = case shown="真" w340 {
              tunnel: w341 -> [_ w342]
              frame #0 {
              }
              frame #1 {
                n270 = stacked-sequence {
                  tunnel: w342 -> [_ w349]
                  frame #0 {
                    w343 = u32 ? ("index")
                    n271 = property on="CameraList 4" class="Ring (严格)"() -> ("Strings []"=w346:string[])  [unwired: 2 in, 2 out]
                    n272 = call "dvp Vi Enum.vi"("unSize"=u32 ?, "index"=w343) -> ("friendlyName out"=w345:string)  [unwired: 8 in, 1 out]
                    n273 = Replace Array Subset ("替换数组子集")(array=w346, new element=w345, index=w343) -> (w347:string[])
                    n274 = property on="CameraList 4" class="Ring (严格)"("Strings []"=w347) -> ()  [unwired: 2 in, 2 out]
                  }
                  frame #1 {
                    n275 = property on="CameraList 4" class="Ring (严格)"() -> ("StringsAndValues[]"=w351:T3)  [unwired: 2 in, 2 out]
                    n276 = Decrement(x=w349) -> (x-1=w348:u32)
                    n277 = for {
                      N: w348 -> [_]
                      shift-right: [w358] -> w350
                      shift-left: w351 -> [w356]
                      i -> [w353]
                      n278 = Increment(x=w353) -> (x+1=w352:i32)
                      n279 = call "dvp Vi Enum.vi"("unSize"=u32 ?, "index"=w352) -> ("friendlyName out"=w359:string)  [unwired: 8 in, 1 out]
                      n280 = To Unsigned Word Integer(number=w352) -> (unsigned 16bit integer=w355:u16)
                      n281 = Bundle("friendlyName out"=w359, w355) -> (w357:cluster{"friendlyName out":string, u16})  [unwired: 1 in]
                      n282 = Build Array (concatenate) ("创建数组")(w356, w357) -> (w358:T3)
                    }
                    n283 = property on="CameraList 4" class="Ring (严格)"("StringsAndValues[]"=w350) -> ()  [unwired: 2 in, 2 out]
                  }
                }
              }
            }
          }
        }
      }
      event #2 {
        w362 = u32 ? items=["OPEN_OFFLINE", "OPEN_NORMAL"] ("type")
        n284 = event-data() -> ()  [unwired: 1 in, 8 out]
        n285 = property on="CameraList 4" class="Ring (严格)"() -> ("RingText.Text"=w361:string)  [unwired: 2 in, 2 out]
        n286 = local write "CloseFlg 4"(i32 ? ("CloseFlg")) -> ()
        n287 = call "dvp Vi Open By Name.vi"("type"=w362, "friendlyName"=w361) -> ("pHandle out"=w364:u32, "function return"=w363:u32)  [unwired: 7 in, 1 out]
        n288 = case shown="1" w363 {
          tunnel: w364 -> [_ w368]
          frame #0 {
            n289 = One Button Dialog(message=string ? ("消息")) -> ()  [unwired: 1 in, 1 out]
          }
          frame #1 {
            n290 = local write "CloseFlg 4"(i32 ? ("CloseFlg")) -> ()
            n291 = call "dvp Vi Start.vi"("handle"=w368) -> ("function return"=w366:u32)  [unwired: 10 in]
            n292 = local write "handle 4"(w368) -> ()
            n293 = case shown="1" w366 {
              tunnel: w368 -> [w372 w384]
              frame #0 {
                w371 = T2 ? ("禁用")
                n294 = local write "handle 4"(u32 ? ("handle")) -> ()
                n295 = local write "CloseFlg 4"(i32 ? ("CloseFlg")) -> ()
                n296 = call "dvp Vi Close.vi"("handle"=w372) -> ()  [unwired: 10 in, 1 out]
                n297 = property on="Set 4" class="Bool"("DisabledEnum"=w371) -> ()  [unwired: 2 in, 2 out]
                n298 = property on="Close 4" class="Bool"("DisabledEnum"=w371) -> ()  [unwired: 2 in, 2 out]
              }
              frame #1 {
                w379 = T4 ? items=["Grayscale (U8)", "Grayscale (I16)", "Grayscale (SGL)", "Complex (CSG)", "RGB (U32)", "HSL (U32)", "RGB (U64)", "Grayscale (U16)"] ("Image Type")
                w382 = T4 ? items=["Grayscale (U8)", "Grayscale (I16)", "Grayscale (SGL)", "Complex (CSG)", "RGB (U32)", "HSL (U32)", "RGB (U64)", "Grayscale (U16)"] ("Image Type")
                w388 = T2 ? ("禁用")
                n299 = call "dvp Vi Get Image Size.vi"("handle"=w384) -> ("function return"=w383:u32)  [unwired: 10 in]
                n300 = call "IMAQ Create"("Border Size"=i32 ?, "Image Name"=string ?, "Image Type"=w379) -> ("New Image"=w376:T1, "error out"=w375:errorcluster)  [unwired: 2 in]
                n301 = call "IMAQ Create"("Border Size"=i32 ?, "Image Name"=string ?, "Image Type"=w382) -> ("New Image"=w374:T1, "error out"=w373:errorcluster)  [unwired: 2 in]
                n302 = Initialize Array(u8 ? ("元素"), w383) -> (w385:u8[])
                n303 = while {
                  shift-right: [w399] -> _
                  shift-left: w384 -> [w399]
                  tunnel: w385 -> [w398]
                  tunnel: w376 -> [w392]
                  tunnel: w375 -> [w391]
                  tunnel: w374 -> [w390]
                  tunnel: w373 -> [w389]
                  stop <- w401 stop-if-true
                  n304 = call "dvp Vi Get Image Data.vi"("handle"=w399, "pbuffer"=w398) -> ("piHeight out"=w396:i32, "function return"=w393:bool, "pformat out"=w394:i32, "pbuffer out"=w395:u32[], "piWidth out"=w397:i32)  [unwired: 9 in]
                  n305 = event shown="[2] \"Set 4\": 鼠标按下" {
                    selector: _ -> [_ _ _]
                    dyn-events: _ -> [_ _ _]
                    timeout: i32 ? -> [_ _ _]
                    tunnel: w399 -> [w428 _ w435]
                    event #0 {
                      n306 = event-data() -> ()  [unwired: 1 in, 5 out]
                      n307 = call "dvp Vi Stop.vi"("handle"=w428) -> ("function return"=w429:u32)  [unwired: 10 in]
                      n308 = case shown="1" w429 {
                        tunnel: w428 -> [_ w432]
                        frame #0 {
                        }
                        frame #1 {
                          w431 = T2 ? ("禁用")
                          n309 = call "dvp Vi Close.vi"("handle"=w432) -> ()  [unwired: 10 in, 1 out]
                          n310 = local write "handle 4"(u32 ? ("handle")) -> ()
                          n311 = property on="Open 4" class="Bool"("DisabledEnum"=T2 ? ("禁用")) -> ()  [unwired: 2 in, 2 out]
                          n312 = local write "CloseFlg 4"(i32 ? ("CloseFlg")) -> ()
                          n313 = property on="Close 4" class="Bool"("DisabledEnum"=w431) -> ()  [unwired: 2 in, 2 out]
                          n314 = property on="Set 4" class="Bool"("DisabledEnum"=w431) -> ()  [unwired: 2 in, 2 out]
                        }
                      }
                    }
                    event #1 {
                      n315 = event-data() -> ()  [unwired: 1 in, 3 out]
                    }
                    event #2 {
                      n316 = event-data() -> ()  [unwired: 1 in, 8 out]
                      n317 = call "dvp Vi Show Property Modal Dialog.vi"("handle"=w435) -> ()  [unwired: 10 in, 1 out]
                    }
                  }
                  n318 = case shown="真" w393 {
                    tunnel: w397 -> [_ w411]
                    tunnel: w396 -> [_ w410]
                    tunnel: w395 -> [_ w408]
                    tunnel: w394 -> [_ w407]
                    tunnel: w392 -> [_ w406]
                    tunnel: w391 -> [_ w405]
                    tunnel: w390 -> [_ w404]
                    tunnel: w389 -> [_ w403]
                    frame #0 {
                    }
                    frame #1 {
                      n319 = case shown="0, 默认" w407 {
                        tunnel: w410 -> [w420 w426]
                        tunnel: w411 -> [w419 w427]
                        tunnel: [w418 w424] -> w409
                        tunnel: w408 -> [w415 w423]
                        tunnel: w406 -> [_ w422]
                        tunnel: w405 -> [_ w421]
                        tunnel: w404 -> [w413 _]
                        tunnel: w403 -> [w412 _]
                        frame #0 {
                          n320 = Type Cast(type=u8[] ?, x=w415) -> (*(type *) &x=w414:u8[])
                          n321 = Reshape Array ("重排数组维数")(w414, w420, w419) -> (w417:u8[][])
                          n322 = call "IMAQ ArrayToImage"("error in (no error)"=w412, "Image Pixels (U8)"=w417, "Image"=w413) -> ("Image Out"=w418:T1)  [unwired: 7 in, 1 out]
                        }
                        frame #1 {
                          n323 = Reshape Array ("重排数组维数")(w423, w426, w427) -> (w425:u32[][])
                          n324 = call "IMAQ ArrayToColorImage"("Image Pixels (U32)"=w425, "Image"=w422, "error in (no error)"=w421) -> ("Image Out"=w424:T1)  [unwired: 2 in, 1 out]
                        }
                      }
                      "Image 4" <- w409
                    }
                  }
                  n325 = local read "CloseFlg 4"() -> (w400:i32)
                  n326 = Equal To 0?(x=w400) -> (x = 0?=w401:bool)
                }
                n327 = property on="Set 4" class="Bool"("DisabledEnum"=w388) -> ()  [unwired: 2 in, 2 out]
                n328 = property on="Close 4" class="Bool"("DisabledEnum"=w388) -> ()  [unwired: 2 in, 2 out]
                n329 = property on="Open 4" class="Bool"("DisabledEnum"=T2 ? ("禁用")) -> ()  [unwired: 2 in, 2 out]
              }
            }
          }
        }
      }
      event #3 {
        n330 = event-data() -> ()  [unwired: 1 in, 4 out]
        n331 = local read "handle 4"() -> (w436:u32)
        n332 = Greater Than 0?(x=w436) -> (x > 0?=w437:bool)
        n333 = case shown="真" w437 {
          tunnel: w436 -> [_ w440]
          frame #0 {
          }
          frame #1 {
            n334 = call "dvp Vi Close.vi"("handle"=w440) -> ()  [unwired: 10 in, 1 out]
            n335 = local write "handle 4"(u32 ? ("handle")) -> ()
          }
        }
        n336 = One Button Dialog(message=string ? ("消息")) -> ()  [unwired: 1 in, 1 out]
      }
    }
  }
  "handle" <- u32 ? ("handle")
  "handle 2" <- u32 ? ("handle")
  "handle 3" <- u32 ? ("handle")
  "handle 4" <- u32 ? ("handle")
